vi "Send_Get_8Bits.vi"(8 "error in (no error)":errorcluster, 10 "Channel":u8, 11 "Simulated uC in":refnum<class "Simulated uC.lvclass">) -> (0 "error out":errorcluster, 2 "Response":string, 3 "Simulated uC out":refnum<class "Simulated uC.lvclass">)   [LabVIEW 2019, in "Simulated uC.lvclass"]
uses:
  Simulated uC.lvclass
  Clase Padre/Marca.ctl
  Clase Padre/Serial Device.lvclass
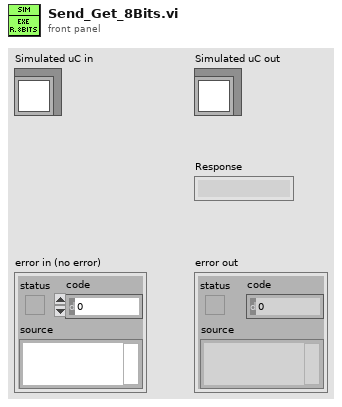
[diagram p1: front panel]
types:
  T1 = typedef "Marca.ctl" = string
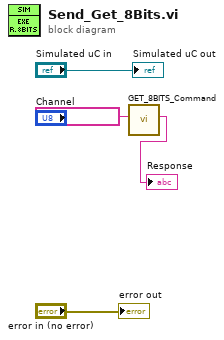
[diagram p0: block diagram]
diagram:
  n1 = call "GET_8BITS_Command.vi"("Marca"=T1 "S") -> ("Expected Response"=→"Response":string)  [unwired: 7 in, 3 out]
  "error out" <- "error in (no error)"
  "Simulated uC out" <- "Simulated uC in"
